vi "kloehn V6 - Open Comm .vi"(8 "error in":errorcluster, 10 "Serial Parameters":T1={"baud rate (9600)"=9600, "data bits (7)"=8, "parity (1:odd)"=enum."None", "stop bits (10: 1 bit)"=10, "flow control (0:none)"=0, "timeout (10sec)"=60000, "termination char"=255, "Enable Termination Char (T)"=TRUE} {"termination char" format="%.0x"; "flow control (0:none)" items=["None"=0, "XON/XOFF"=1, "RTS/CTS"=2, "DTR/DSR"=4]; "stop bits (10: 1 bit)" items=["1.0"=10, "1.5"=15, "2.0"=20]; "data bits (7)" min=5 max=8 step=1}, 11 "VISA Ref":refnum<visa-resource-name>="ASRL1::INSTR") -> (0 "error out":errorcluster, 3 "VISA Ref DUP":refnum<visa-resource-name>)   [LabVIEW 2010]
uses:
  <vilib>/Instr/_visa.llb/VISA Configure Serial Port (Instr).vi
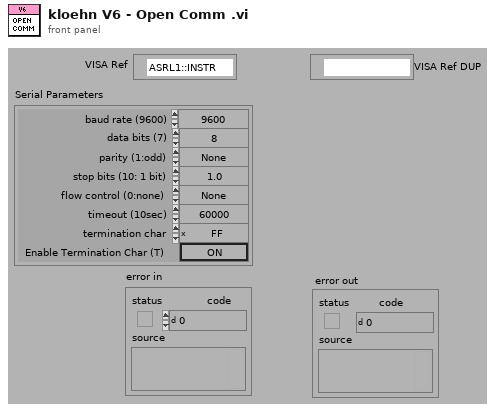
[diagram p1: front panel]
types:
  T1 = cluster{"baud rate (9600)":u32, "data bits (7)":u16, "parity (1:odd)":enum16{"None", "Odd", "Even", "Mark", "Space"}, "stop bits (10: 1 bit)":u16, "flow control (0:none)":u16, "timeout (10sec)":u32, "termination char":u8, "Enable Termination Char (T)":bool}
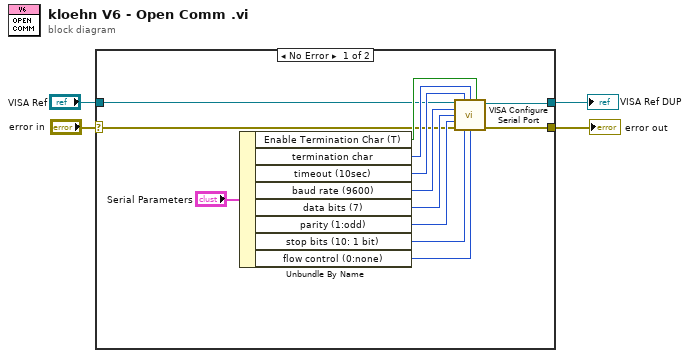
[diagram p0: block diagram]
diagram:
  n1 = case shown="No Error" "error in" {
    selector: "error in" -> [w8 w19]
    tunnel: [w5 w19] -> w4
    tunnel: [w6 w18] -> w2
    tunnel: "VISA Ref" -> [w7 w18]
    frame No Error {
      n2 = Unbundle By Name("Serial Parameters") -> ("Enable Termination Char (T)"=w17:bool, "termination char"=w16:u8, "timeout (10sec)"=w15:u32, "baud rate (9600)"=w10:u32, "data bits (7)"=w11:u16, "parity (1:odd)"=w12:enum16{"None", "Odd", "Even", "Mark", "Space"}, "stop bits (10: 1 bit)"=w13:u16, "flow control (0:none)"=w14:u16)
      n3 = call-poly "VISA Configure Serial Port"("VISA resource name"=w7, "timeout (10sec)"=w15, "termination char\n(0xA = '\\n' = LF)"=w16, "Enable Termination\nChar (T)"=w17, "baud rate (9600)"=w10, "data bits (8)"=w11, "parity (0:none)"=w12, "error in (no error)"=w8, "stop bits (10: 1 bit)"=w13, "flow control (0:none)"=w14) -> ("VISA resource name out"=w6:refnum<visa-resource-name>, "error out"=w5:errorcluster)  [unwired: 4 in]
    }
    frame Error {
    }
  }
  "error out" <- w4
  "VISA Ref DUP" <- w2
